vi "Offset Locking and Active Slave Locking v3.3.vi"() -> ()   [LabVIEW 2018]
uses:
  <vilib>/Utility/error.llb/DialogType.ctl
  <vilib>/measure/mamon.llb/Waveform Peak Detection for 1 Chan.vi
  <vilib>/addons/control/pid/pid.llb/PID Advanced (DBL).vi
  <vilib>/measure/NI_MAPro.lvlib
  <vilib>/addons/control/pid/NI_PID_pid.lvlib
  <vilib>/Analysis/NI_AALBase.lvlib
panel:
  in  "Drift Threshold":dbl=0.98
  out "Master-Slave Peak Height":dbl(graph)
  out "Slave's Current\n Adjustment (V)":dbl
  out "Master-Slave Peak Height":dbl
  in  "Locked Peak\nHeight Min":dbl=0.9
  in  "Active Slave \nLock On?":bool
  in  "Manual Slave Current Adjust":dbl format="%#_g V"
  out "Target \nPeak":dbl
  out "Calibration\n Peaks":dbl[](array[numeric])
  in  "Minimum \namplitude\nfor Calibration":dbl=1.1 format="%#_13g V"
  in  "width":i32=1000
  in  "Minimum \namplitude\nfor Target":dbl=0.6 format="%#_13g V"
  out "Run Time (min)":dbl
  out "# found":i32
  out "Offset":dbl(graph)
  in  "Manual PZT Control":dbl format="%#_g V"
  in  "Engage \nPZT PID ?":bool
  out "Offset (GHz)":dbl format="%#_4g"
  in  "# of Shots for Averaging":i32=100
  in  "Name Convention":string="Chirp Offset Lock Log"
  in  "Save Directory":path=path "C:/Users/LabUser/Google Drive/Measurements/04-2018"
  out "Enough\n peaks?":bool
  out "PZT Output":dbl(graph)
  in  "PID Gains":T1={"proportional gain (Kc)"=-1.0, "integral time (Ti, min)"=0.01, "derivative time (Td, min)"=0.0} {"derivative time (Td, min)" format="%.3f"; "integral time (Ti, min)" format="%.3f"; "proportional gain (Kc)" format="%.3f"}
  out "dt out (s)":dbl format="%.3f"
  in  "Frequency Offset \nSetpoint (GHz)":dbl=4.0 format="%.3f"
  out "GHz/sec":dbl
  out "dt":dbl format="%#_4g"
  out "Peak Locations":dbl[](array[numeric]) format="%.2p"
  out "Peak Amplitudes":dbl[](array[numeric]) format="%.2p"
  out "10 GHz FPI":dynamicdata(graph)
  in  "Stop":bool
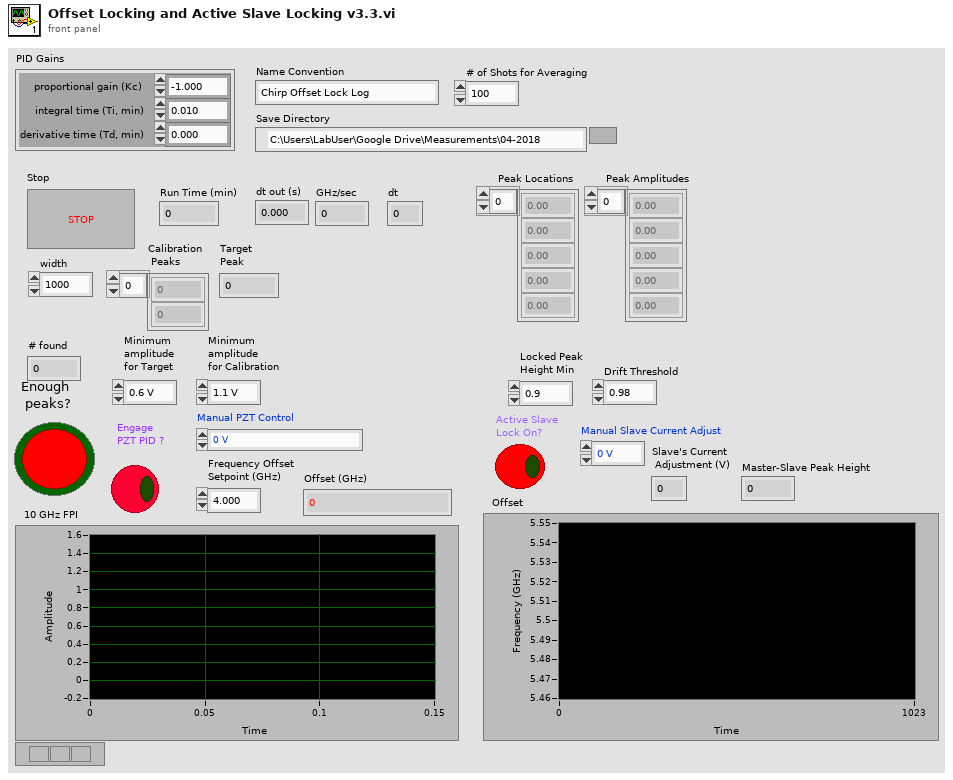
[diagram p1: front panel]
types:
  T1 = cluster{"proportional gain (Kc)":dbl, "integral time (Ti, min)":dbl, "derivative time (Td, min)":dbl}
  T2 = enum8{"Enabled", "Disabled", "Disabled and Grayed Out"}
  T3 = typedef "DialogType.ctl" = u16
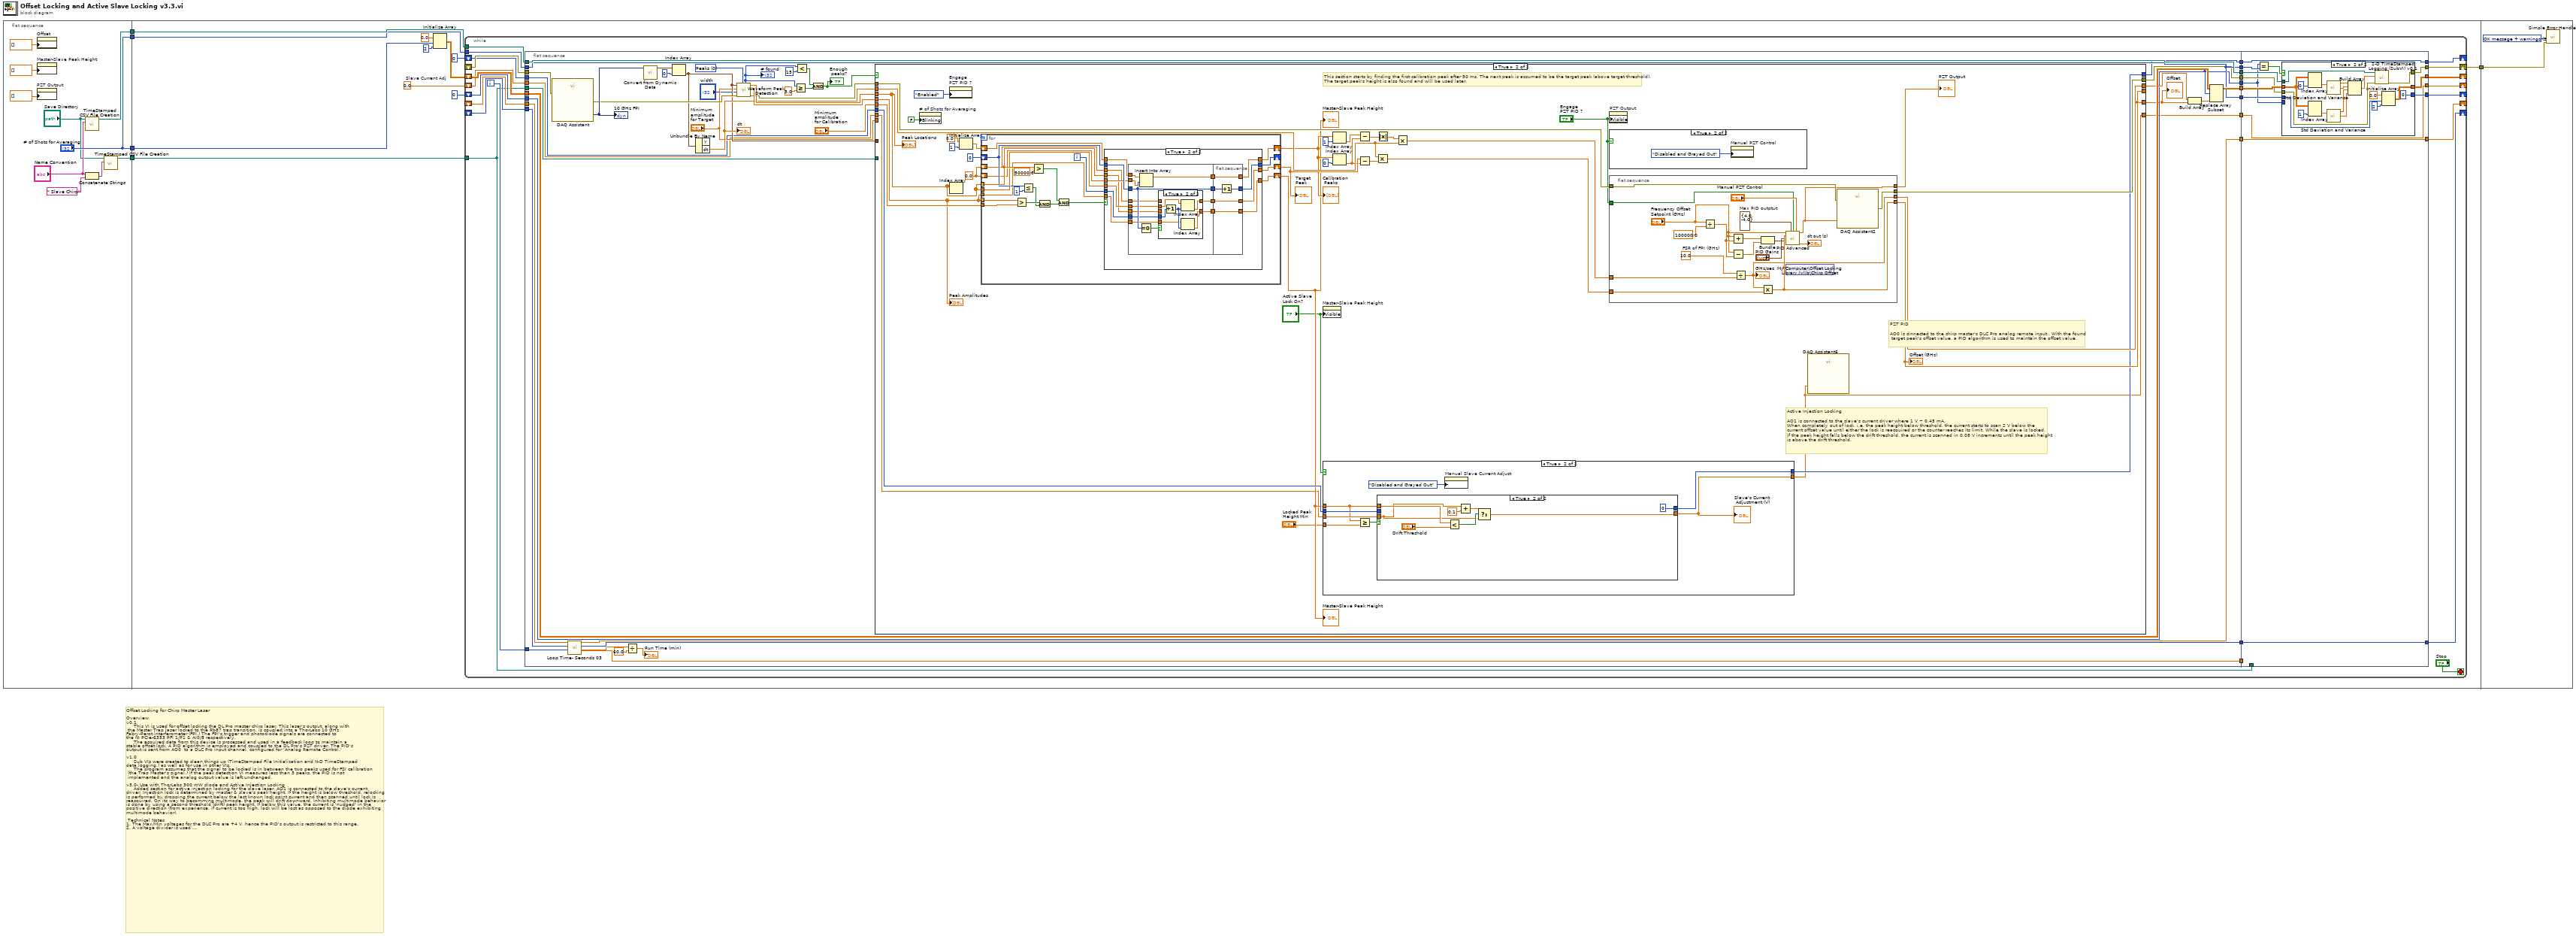
[diagram p0: block diagram]
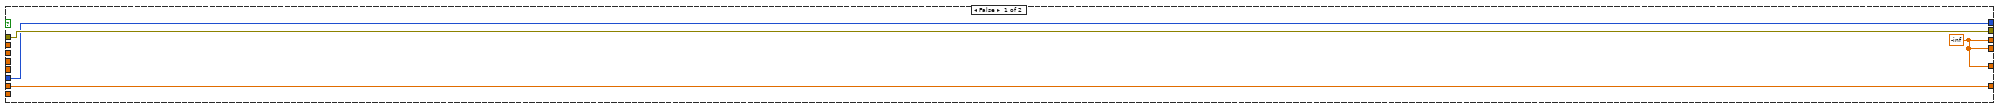
[diagram p2: hidden frame]
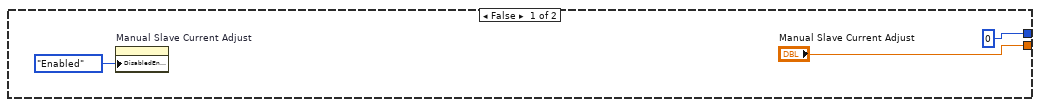
[diagram p3: hidden frame]
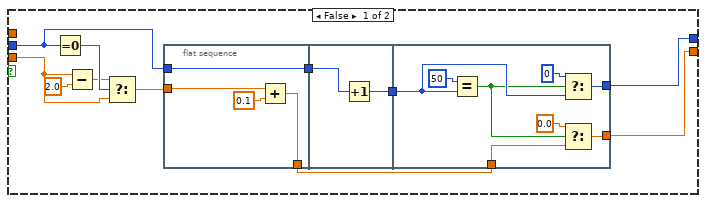
[diagram p4: hidden frame]
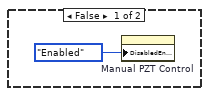
[diagram p5: hidden frame]
diagram:
  # "Offset Locking for Chirp Master Laser\n\nOverview\nv0.1\n     This VI is used for offset locking the DL Pro master chirp laser. This laser's output, along with\n the Master Trap laser locked to the Rb87 trap transition, is coupled into a ThorLabs 10 GHz \nFabry-Perot interferometer (FPI.) The FPI's trigger and photodiode signals are connected to \nthe NI PCIe-6353 PFI 1/P1 & AI0/8 respectively. \n     The acquired data from this device is processed and used in a feedback loop to maintain a \nstable offset lock. A PID algorithm is employed and coupled to the DL Pro's PZT driver. The PID's\noutput is sent from AO0  to a DLC Pro input channel, configured for 'Analog Remote Control.'\n\nv1.0\n     Sub VIs were created to clean things up (TimeStamped File Initialization and N-D TimeStamped \ndata logging,) as well as for use in other VIs.\n     The program assumes that the signal to be locked is in between the two peaks used for FSI calibration\n (the Trap Master's signal.) If the peak detection VI measures less than 3 peaks, the PID is not\n implemented and the analog output value is left unchanged.\n\nv3.0- Use with ThorLabs 300 mW diode and Active Injection Locking\n     Added section for active injection locking for the slave laser. AO1 is connected to the slave's current \ndriver. Injection lock is determined by master & slave's peak height. If the height is below threshold, relocking \nis performed by dropping the current below the last known lock point current and then scanned until lock is \nreacquired. On its way to becomming multimode, the peak will drift downward. Inhibiting multimode behavior\nis done by using a second threshold (drift) peak height. If below this value, the current is 'nudged' in the \npositive direction (from experience, if current is too high, lock will be lost as opposed to the diode exhibiting \nmultimode behavior). \n\n Technical Notes\n1. The Max/Min voltages for the DLC Pro are +4 V, hence the PID's output is restricted to this range.\n2. A voltage divider is used for the AO1 output to the current controller. This restricts the current range to\nabout +/-4.5 mA while using the max +/-10 V range of the AO."
  n1 = flat-sequence {
    tunnel: [w15] -> w5
    tunnel: ["# of Shots for Averaging"] -> w3
    tunnel: ["# of Shots for Averaging"] -> w2
    tunnel: [w7] -> w1
    tunnel: w5 -> [w26]
    tunnel: [w25] -> w4
    tunnel: w3 -> [w23]
    tunnel: w2 -> [w20]
    tunnel: w1 -> [w18]
    tunnel: w4 -> [w304]
    frame #0 {
      n2 = property on="Offset" class="WFChart (strict)"("History Data"=dbl[] []) -> ()  [unwired: 2 in, 2 out]
      n3 = property on="Master-Slave Peak Height" class="WFChart (strict)"("History Data"=dbl[] []) -> ()  [unwired: 2 in, 2 out]
      n4 = property on="PZT Output" class="WFChart (strict)"("History Data"=dbl[] []) -> ()  [unwired: 2 in, 2 out]
      n5 = call "TimeStamped CSV File Creation.vi"("Name Convention"="Name Convention", "Save Directory"="Save Directory") -> ("path"=w15:path)  [unwired: 8 in, 1 out]
      n6 = Concatenate Strings("Name Convention", " Slave Chirp" ("string")) -> (w9:string)
      n7 = call "TimeStamped CSV File Creation.vi"("Name Convention"=w9, "Save Directory"="Save Directory") -> ("path"=w7:path)  [unwired: 8 in, 1 out]
    }
    frame #1 {
      w17 = 0.0  # Slave Current Adj
      n8 = Initialize Array(0.0 ("element"), w20, 2 ("dimension size")) -> (w22:dbl[][])
      n9 = while {
        shift-right: [w44] -> w25
        shift-left: _ -> [w55]
        tunnel: w26 -> [w53]
        shift-right: [w42] -> _
        shift-left: 0 -> [w51]
        tunnel: w23 -> [w49]
        shift-right: [w43] -> _
        shift-left: w22 -> [w46]
        shift-right: [w40] -> _
        shift-left: _ -> [w37]
        shift-right: [w38] -> _
        shift-left: _ -> [w36]
        tunnel: w18 -> [w33]
        shift-right: [w30] -> _
        shift-left: w17 -> [w32]
        shift-right: [w27] -> _
        shift-left: 0 -> [w29]
        i -> [w35]
        stop <- "Stop" stop-if-true
        n10 = flat-sequence {
          tunnel: w55 -> [w90]
          tunnel: [w66] -> w54
          tunnel: w53 -> [w88]
          tunnel: [w88] -> w52
          tunnel: w51 -> [w82]
          tunnel: [w82] -> w50
          tunnel: w49 -> [w83]
          tunnel: [w83] -> w48
          tunnel: [w87] -> w47
          tunnel: w46 -> [w86]
          tunnel: [w83] -> w45
          tunnel: [w81] -> w41
          tunnel: [w80] -> w39
          tunnel: w37 -> [w79]
          tunnel: w36 -> [w78]
          tunnel: w35 -> [w77]
          tunnel: [w69] -> w34
          tunnel: w33 -> [w64]
          tunnel: w32 -> [w60]
          tunnel: [w59] -> w31
          tunnel: w29 -> [w58]
          tunnel: [w57] -> w28
          tunnel: w54 -> [w277]
          tunnel: w52 -> [w278]
          tunnel: w50 -> [w272]
          tunnel: w48 -> [w282]
          tunnel: w47 -> [w279]
          tunnel: w45 -> [w280]
          tunnel: [w271] -> w44
          tunnel: [w276] -> w43
          tunnel: [w275] -> w42
          tunnel: w41 -> [w274]
          tunnel: [w274] -> w40
          tunnel: [w273] -> w38
          tunnel: w39 -> [w273]
          tunnel: w34 -> [_]
          tunnel: w33 -> [_]
          tunnel: w31 -> [w270]
          tunnel: [w270] -> w30
          tunnel: w28 -> [w269]
          tunnel: [w269] -> w27
          frame #0 {
            w92 = u16 0 items=["Peaks", "Valleys"] ("peaks/valleys")
            n11 = call "DAQ Assistant"("error in"=w90) -> ("data"=w96:dynamicdata, "error out"=w89:errorcluster)  [unwired: 16 in, 1 out]
            "10 GHz FPI" <- w96
            n12 = call "Loop Time- Seconds 03.vi"("Loop Iteration"=w77, "Shift Registered Time In"=w78, "Shift Registered In"=w79) -> ("t"=w69:dbl, "Shift Registered Time Out"=w80:u32, "Shift Registered Out"=w81:dbl)  [unwired: 6 in]
            n13 = Divide(x=w69, y=60.0) -> (x/y=→"Run Time (min)":dbl)
            n14 = call "Convert from Dynamic Data"("Dynamic Data Type"=w96) -> ("Array of Waveform"=w98:waveform(dbl)[])  [unwired: 3 in]
            n15 = Index Array(array=w98, index=0) -> (element=w65:waveform(dbl))
            n16 = Unbundle By Name(w65) -> ("dt"=w93:dbl)  [unwired: 1 out]
            "dt" <- w93
            n17 = call-poly <vilib>:"Waveform Peak Detection.vi"("peaks/valleys"=w92, "error in"=w89, "width"="width", "threshold"="Minimum \namplitude\nfor Target", "Signal In"=w65) -> ("error out"=w67:errorcluster, "Amplitudes"=w95:dbl[], "Locations"=w94:dbl[], "# found"=w74:i32)  [unwired: 2 in, 1 out]
            "# found" <- w74
            n18 = Greater Or Equal?(x=w74, y=3.0) -> (x >= y?=w75:bool)
            n19 = Less?(x=w74, y=15) -> (x < y?=w72:bool)
            n20 = And(x=w72, y=w75) -> (x .and. y?=w71:bool)
            "Enough\n peaks?" <- w71
            n21 = case shown="True" w71 {
              tunnel: w95 -> [_ w114]
              tunnel: w94 -> [_ w122]
              tunnel: w93 -> [_ w133]
              tunnel: [w102 w128] -> w85
              tunnel: [w102 w129] -> w76
              tunnel: [w102 w129] -> _
              tunnel: w67 -> [w101 w131]
              tunnel: [w101 w130] -> w66
              tunnel: w65 -> [_ _]
              tunnel: "Minimum \namplitude\nfor Target" -> [_ _]
              tunnel: w64 -> [_ _]
              tunnel: "Minimum \namplitude\nfor Calibration" -> [_ w127]
              tunnel: w60 -> [w100 w103]
              tunnel: [w100 w104] -> w59
              tunnel: w58 -> [w99 w113]
              tunnel: [w99 w112] -> w57
              frame False {
                w102 = -inf
              }
              frame True {
                w115 = 0.0
                # "PZT PID\n\nAO0 is cinnected to the chirp master's DLC Pro analog remote input . With the found\n target peak's offset value, a PID algorithm is used to maintain the offset value."
                # "Active Injection Locking \n\nAO1 is connected to the slave's current driver where 1 V ~ 0.45 mA. \nWhen completely out of lock, i.e. the peak height below threshold, the current starts to scan 2 V below the\ncurrent offset value until either the lock is reacquired or the counter reaches its limit. While the slave is locked, \nif the peak height falls below the drift threshold, the current is scanned in 0.08 V increments until the peak height \nis above the drift threshold."
                # "This section starts by finding the first calibration peak after 50 ms. The next peak is assumed to be the target peak (above target threshold).\nThe target peak's height is also found and will be used later."
                n22 = property on="# of Shots for Averaging" class="DigNum (strict)"("Blinking"=FALSE) -> ()  [unwired: 2 in, 2 out]
                n23 = property on="Engage \nPZT PID ?" class="Bool (strict)"("DisabledEnum"=T2."Enabled" ("Disabled")) -> ()  [unwired: 2 in, 2 out]
                n24 = Index Array(array=w122) -> ()  [unwired: 1 in, 1 out]
                n25 = Initialize Array(0.0 ("element"), 1 ("dimension size")) -> (w123:dbl[])
                n26 = for {
                  tunnel: w122 -> [w213] mode=indexing
                  tunnel: w114 -> [w206] mode=indexing
                  tunnel: w127 -> [w218]
                  shift-right: [w209] -> w121
                  shift-left: w123 -> [w223]
                  shift-right: [w222] -> _
                  shift-left: 0 -> [w210]
                  shift-right: [w208] -> w117
                  shift-left: w115 -> [w207]
                  tunnel: w122 -> [w211]
                  shift-right: [w204] -> w111
                  shift-left: w115 -> [w205]
                  tunnel: w114 -> [w203]
                  i -> [w212]
                  n27 = Greater?(x=w206, y=w218) -> (0:w221:bool)
                  n28 = Less Or Equal?(x=w210, y=1) -> (x <= y?=w219:bool)
                  n29 = Greater?(x=w213, y=50000.0) -> (0:w216:bool)
                  n30 = And(x=w221, y=w219) -> (x .and. y?=w217:bool)
                  n31 = And(x=w216, y=w217) -> (x .and. y?=w214:bool)
                  n32 = case shown="True" w214 {
                    tunnel: w223 -> [w226 w243]
                    tunnel: w210 -> [w227 w242]
                    tunnel: [w227 w239] -> w222
                    tunnel: w213 -> [_ w241]
                    tunnel: w212 -> [_ w236]
                    tunnel: w211 -> [_ w235]
                    tunnel: [w226 w237] -> w209
                    tunnel: [w225 w233] -> w208
                    tunnel: w207 -> [w225 w232]
                    tunnel: w205 -> [w224 w231]
                    tunnel: [w224 w228] -> w204
                    tunnel: w203 -> [_ w230]
                    frame False {
                    }
                    frame True {
                      n33 = flat-sequence {
                        tunnel: w243 -> [w255]
                        tunnel: w242 -> [w252]
                        tunnel: w241 -> [w254]
                        tunnel: [w253] -> w240
                        tunnel: [w252] -> w238
                        tunnel: w236 -> [w249]
                        tunnel: w235 -> [w251]
                        tunnel: [w250] -> w234
                        tunnel: w232 -> [w247]
                        tunnel: w231 -> [w244]
                        tunnel: w230 -> [w246]
                        tunnel: [w245] -> w229
                        tunnel: w240 -> [w266]
                        tunnel: [w268] -> w239
                        tunnel: w238 -> [w267]
                        tunnel: [w266] -> w237
                        tunnel: w234 -> [w265]
                        tunnel: [w265] -> w233
                        tunnel: w229 -> [w264]
                        tunnel: [w264] -> w228
                        frame #0 {
                          n34 = Equal To 0?(x=w252) -> (x = 0?=w248:bool)
                          n35 = Insert Into Array(array=w255, index=w252, new element=w254) -> (w253:dbl[])
                          n36 = case shown="True" w248 {
                            tunnel: w251 -> [_ w263]
                            tunnel: [w257 w262] -> w250
                            tunnel: w249 -> [_ w261]
                            tunnel: w247 -> [w257 _]
                            tunnel: w246 -> [_ w259]
                            tunnel: [w256 w258] -> w245
                            tunnel: w244 -> [w256 _]
                            frame False {
                            }
                            frame True {
                              n37 = Increment(x=w261) -> (x+1=w260:i32)
                              n38 = Index Array(array=w263, index=w260) -> (element=w262:dbl)
                              n39 = Index Array(array=w259, index=w260) -> (element=w258:dbl)
                            }
                          }
                        }
                        frame #1 {
                          n40 = Increment(x=w267) -> (x+1=w268:i32)
                        }
                      }
                    }
                  }
                }
                "Calibration\n Peaks" <- w121
                "Target \nPeak" <- w117
                "Master-Slave Peak Height" <- w111
                "Master-Slave Peak Height" <- w111
                n41 = property on="Master-Slave Peak Height" class="WFChart (strict)"("Visible"="Active Slave \nLock On?") -> ()  [unwired: 2 in, 2 out]
                n42 = case shown="True" "Active Slave \nLock On?" {
                  tunnel: ["Manual Slave Current Adjust" w161] -> w104
                  tunnel: "Locked Peak\nHeight Min" -> [_ w165]
                  tunnel: w111 -> [_ w162]
                  tunnel: w103 -> [_ w166]
                  tunnel: w113 -> [_ w164]
                  tunnel: [0 ("t") w163] -> w112
                  frame False {
                    n43 = property on="Manual Slave Current Adjust" class="DigNum (strict)"("DisabledEnum"=T2."Enabled" ("Disabled")) -> ()  [unwired: 2 in, 2 out]
                  }
                  frame True {
                    n44 = Greater Or Equal?(x=w162, y=w165) -> (x >= y?=w167:bool)
                    n45 = case shown="True" w167 {
                      tunnel: w166 -> [w171 w195]
                      tunnel: [w169 w196] -> w161
                      tunnel: w164 -> [w174 _]
                      tunnel: [w175 0 ("t")] -> w163
                      tunnel: w162 -> [_ w199]
                      frame False {
                        n46 = Equal To 0?(x=w174) -> (x = 0?=w173:bool)
                        n47 = Subtract(x=w171, y=2.0) -> (x-y=w172:dbl)
                        n48 = Select(t=w172, s=w173, f=w171) -> (s? t:f=w170:dbl)
                        n49 = flat-sequence {
                          tunnel: w170 -> [w182]
                          tunnel: w174 -> [w180]
                          tunnel: [w181] -> w168
                          tunnel: [w180] -> w177
                          tunnel: w177 -> [w184]
                          tunnel: [w183] -> w176
                          tunnel: w176 -> [w191]
                          tunnel: [w189] -> w175
                          tunnel: w168 -> [w187]
                          tunnel: [w186] -> w169
                          frame #0 {
                            n50 = Add(x=w182, y=0.1 ("x")) -> (x+y=w181:dbl)
                          }
                          frame #1 {
                            n51 = Increment(x=w184) -> (x+1=w183:i32)
                          }
                          frame #2 {
                            n52 = Equal?(x=50, y=w191) -> (x = y?=w188:bool)
                            n53 = Select(t=0, s=w188, f=w191) -> (s? t:f=w189:i32)
                            n54 = Select(t=0.0, s=w188, f=w187) -> (s? t:f=w186:dbl)
                          }
                        }
                      }
                      frame True {
                        n55 = Less?(x=w199, y="Drift Threshold") -> (x < y?=w197:bool)
                        n56 = Add(x=w195, y=0.1) -> (x+y=w193:dbl)
                        n57 = Select(t=w193, s=w197, f=w195) -> (s? t:f=w196:dbl)
                      }
                    }
                    "Slave's Current\n Adjustment (V)" <- w161
                    n58 = property on="Manual Slave Current Adjust" class="DigNum (strict)"("DisabledEnum"=T2."Disabled and Grayed Out" ("Disabled")) -> ()  [unwired: 2 in, 2 out]
                  }
                }
                n59 = Index Array(array=w121, index=1) -> (element=w118:dbl)
                n60 = Index Array(array=w121, index=0) -> (element=w116:dbl)
                n61 = Subtract(x=w118, y=w116) -> (x-y=w136:dbl)
                n62 = Subtract(x=w117, y=w116) -> (x-y=w134:dbl)
                n63 = Multiply(x=w133, y=w134) -> (x*y=w132:dbl)
                n64 = Absolute Value(x=w136) -> (abs(x)=w135:dbl)
                n65 = Multiply(x=w135, y=w133) -> (x*y=w137:dbl)
                n66 = property on="PZT Output" class="WFChart (strict)"("Visible"="Engage \nPZT PID ?") -> ()  [unwired: 2 in, 2 out]
                n67 = case shown="True" "Engage \nPZT PID ?" {
                  frame False {
                    n68 = property on="Manual PZT Control" class="DigNum (strict)"("DisabledEnum"=T2."Enabled" ("Disabled")) -> ()  [unwired: 2 in, 2 out]
                  }
                  frame True {
                    n69 = property on="Manual PZT Control" class="DigNum (strict)"("DisabledEnum"=T2."Disabled and Grayed Out" ("Disabled")) -> ()  [unwired: 2 in, 2 out]
                  }
                }
                n70 = flat-sequence {
                  tunnel: w137 -> [w155]
                  tunnel: w132 -> [w154]
                  tunnel: w131 -> [w153]
                  tunnel: [w152] -> w130
                  tunnel: [w151] -> w129
                  tunnel: [w150] -> w128
                  tunnel: [w145] -> w110
                  tunnel: "Engage \nPZT PID ?" -> [w144]
                  frame #0 {
                    w147 = cluster{"output high":dbl, "output low":dbl} {"output high"=4.0, "output low"=-4.0}  # Max PID outptut
                    w156 = 10.0  # FSR of FPI (GHz)
                    n71 = Divide(x="Frequency Offset \nSetpoint (GHz)", y=100000.0) -> (x/y=w142:dbl)
                    n72 = Add(x="Frequency Offset \nSetpoint (GHz)", y=w142) -> (x+y=w140:dbl)
                    n73 = Subtract(x="Frequency Offset \nSetpoint (GHz)", y=w142) -> (x-y=w139:dbl)
                    n74 = Divide(x=w156, y=w155) -> (x/y=w150:dbl)
                    "GHz/sec" <- w150
                    n75 = Bundle(w140, w139) -> (w138:cluster{dbl, dbl})  [unwired: 1 in]
                    n76 = Multiply(x=w150, y=w154) -> (x*y=w151:dbl)
                    n77 = call-poly <vilib>:"PID Advanced.vi"("setpoint"="Frequency Offset \nSetpoint (GHz)", "output range"=w147, "auto? (T)"=w144, "manual control"="Manual PZT Control", "process variable"=w151, "setpoint range"=w138, "PID gains"="PID Gains") -> ("output"=w145:dbl, "dt out (s)"=→"dt out (s)":dbl)  [unwired: 7 in]
                    n78 = shared-variable "My Computer\\Offset Locking Library.lvlib\\Chirp Offset"(w151) -> ()  [unwired: 1 in, 1 out]
                    n79 = call "DAQ Assistant2"("data"=w145, "error in"=w153) -> ("error out"=w152:errorcluster)  [unwired: 16 in, 1 out]
                  }
                }
                n80 = call "DAQ Assistant6"("data"=w104) -> ()  [unwired: 17 in, 2 out]
                "Peak Amplitudes" <- w114
                "Peak Locations" <- w122
                "Offset (GHz)" <- w129
                "PZT Output" <- w110
              }
            }
            "Offset" <- w76
            n81 = Build Array(w85, w76) -> (w84:dbl[])
            n82 = Replace Array Subset(array=w86, new element=w84, index (row)=w82) -> (w87:dbl[][])  [unwired: 1 in]
          }
          frame #1 {
            n83 = Equal?(x=w272, y=w282) -> (x = y?=w281:bool)
            n84 = case shown="True" w281 {
              tunnel: w280 -> [_ w286]
              tunnel: w279 -> [w285 w299]
              tunnel: w278 -> [_ w293]
              tunnel: w277 -> [w283 w292]
              tunnel: [w285 w289] -> w276
              tunnel: w272 -> [w284 _]
              tunnel: [w284 0] -> w275
              tunnel: [w283 w287] -> w271
              frame False {
              }
              frame True {
                n85 = Index Array(array=w299, index (col)=0 ("disabled index (col)")) -> (element=w302:dbl[])  [unwired: 1 in]
                n86 = Index Array(array=w299, index (col)=1 ("disabled index (col)")) -> (element=w300:dbl[])  [unwired: 1 in]
                n87 = call <vilib>:"Std Deviation and Variance.vi"("X"=w302) -> ("mean"=w298:dbl, "standard deviation"=w297:dbl)  [unwired: 1 in, 1 out]
                n88 = call <vilib>:"Std Deviation and Variance.vi"("X"=w300) -> ("mean"=w296:dbl, "standard deviation"=w295:dbl)  [unwired: 1 in, 1 out]
                n89 = Build Array(w298, w297, w296, w295) -> (w294:dbl[])
                n90 = call "2-D TimeStamped Logging (SubVI) v0.1.vi"("error in (no error)"=w292, "array"=w294, "path"=w293) -> ("error out"=w287:errorcluster)  [unwired: 8 in]
                n91 = Initialize Array(0.0 ("element"), w286, 2 ("dimension size")) -> (w289:dbl[][])
              }
            }
          }
        }
      }
    }
    frame #2 {
      w305 = T3 3 items=["no dialog", "OK message", "continue or stop message", "OK message + warnings", "continue/stop + warnings"] ("type of dialog (OK msg:1)")
      n92 = call <vilib>:"Simple Error Handler.vi"("type of dialog (OK msg:1)"=w305, "error in (no error)"=w304) -> ()  [unwired: 3 in, 5 out]
    }
  }
